vi "RVHR - Coerce Slider.vi"(6 "Local Data in":T1, 7 "UI Refs":T8, 8 "error in (no error)":errorcluster, 11 "New Distance":dbl) -> (0 "error out":errorcluster, 3 "Coerced Distance":dbl, 4 "Local Data out":T1)   [LabVIEW 2024]
uses:
  Controls/RVHR - UI Refs.ctl
  Controls/RVHR - Local Data.ctl
  Controls/Test Cluster.ctl
  Controls/Excluded Information.ctl
  Controls/Language.ctl
  Controls/Device_Type.ctl
  <vilib>/Utility/miscctls.llb/LVRectTypeDef.ctl
  <vilib>/Utility/miscctls.llb/LVBoundsTypeDef.ctl
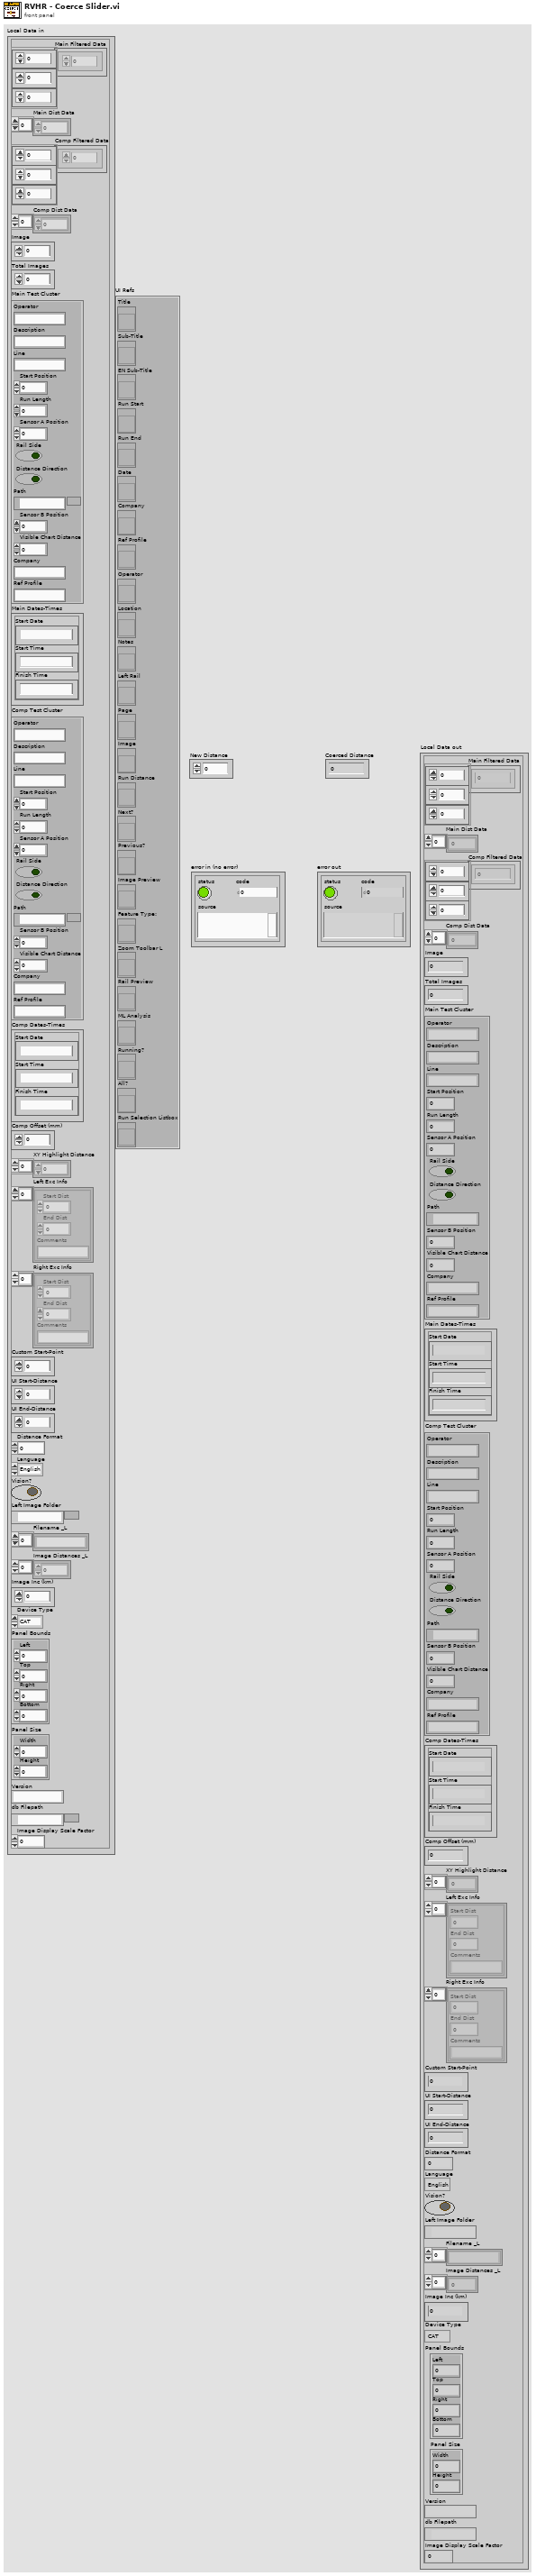
[diagram p1: front panel]
types:
  T1 = typedef "RVHR - Local Data.ctl" = cluster{"Main Filtered Data":dbl[][][], "Main Dist Data":dbl[], "Comp Filtered Data":dbl[][][], "Comp Dist Data":dbl[], "Image":u16, "Total Images":u16, "Main Test Cluster":T2, "Main Dates-Times":cluster{"Start Date":string, "Start Time":string, "Finish Time":string}, "Comp Test Cluster":T2, "Comp Dates-Times":cluster{"Start Date":string, "Start Time":string, "Finish Time":string}, "Comp Offset (mm)":i64, "XY Highlight Distance":dbl[], "Left Exc Info":T3[], "Right Exc Info":T3[], "Custom Start-Point":dbl, "UI Start-Distance":dbl, "UI End-Distance":dbl, "Distance Format":u8, "Language":T4, "Vision?":bool, "Left Image Folder":path, "Filename _L":string[], "Image Distances _L":dbl[], "Image Inc (km)":dbl, "Device Type":T5, "Panel Bounds":T6, "Panel Size":T7, "Version":string, "db Filepath":path, "Image Display Scale Factor":dbl}
  T2 = typedef "Test Cluster.ctl" = cluster{"Operator":string, "Description":string, "Line":string, "Start Position":dbl, "Run Length":dbl, "Sensor A Position":dbl, "Rail Side":bool, "Distance Direction":bool, "Path":path, "Sensor B Position":dbl, "Visible Chart Distance":dbl, "Company":string, "Ref Profile":string}
  T3 = typedef "Excluded Information.ctl" = cluster{"Start Dist":dbl, "End Dist":dbl, "Comments":string}
  T4 = typedef "Language.ctl" = enum16{"English", "Chinese", "German"}
  T5 = typedef "Device_Type.ctl" = enum16{"CAT", "Bi-CAT", "YRCA", "RCA", "RV-HR", "TV-HR"}
  T6 = typedef "LVRectTypeDef.ctl" = cluster{"Left":i16, "Top":i16, "Right":i16, "Bottom":i16}
  T7 = typedef "LVBoundsTypeDef.ctl" = cluster{"Width":u32, "Height":u32}
  T8 = typedef "RVHR - UI Refs.ctl" = cluster{"Title":refnum<vi>, "Sub-Title":refnum<vi>, "EN Sub-Title":refnum<vi>, "Run Start":refnum<vi>, "Run End":refnum<vi>, "Date":refnum<vi>, "Company":refnum<vi>, "Ref Profile":refnum<vi>, "Operator":refnum<vi>, "Location":refnum<vi>, "Notes":refnum<vi>, "Left Rail":refnum<vi>, "Page":refnum<vi>, "Image":refnum<vi>, "Run Distance":refnum<vi>, "Next?":refnum<vi>, "Previous?":refnum<vi>, "Image Preview":refnum<vi>, "Feature Type:":refnum<vi>, "Zoom Toolbar L":refnum<vi>, "Rail Preview":refnum<vi>, "ML Analysis":refnum<vi>, "Running?":refnum<vi>, "All?":refnum<vi>, "Run Selection Listbox":refnum<vi>}
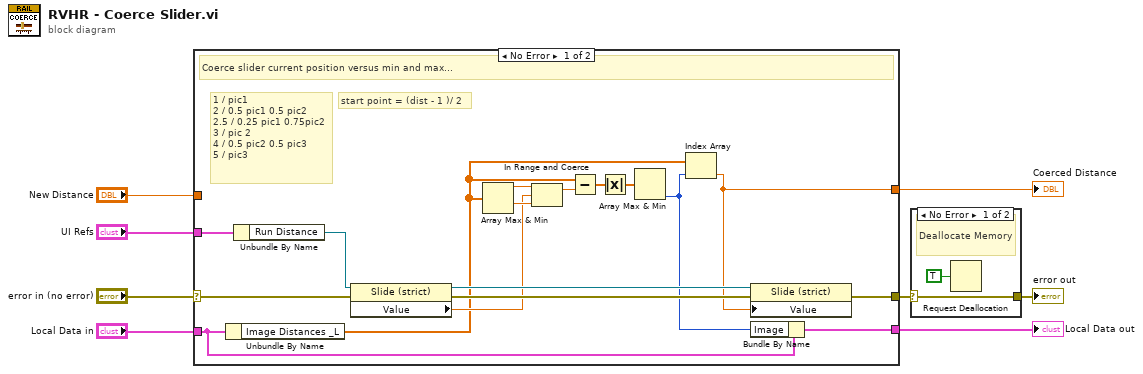
[diagram p0: block diagram]
diagram:
  n1 = case shown="No Error" "error in (no error)" {
    selector: "error in (no error)" -> [w24 w27]
    tunnel: "UI Refs" -> [w25 _]
    tunnel: [w20 w27] -> w3
    tunnel: [w12 _] -> w8
    tunnel: "New Distance" -> [_ _]
    tunnel: "Local Data in" -> [w11 w26]
    tunnel: [w9 w26] -> w1
    frame No Error {
      # "start point = (dist - 1 )/ 2"
      # "1 / pic1\n2 / 0.5 pic1 0.5 pic2\n2.5 / 0.25 pic1 0.75pic2\n3 / pic 2\n4 / 0.5 pic2 0.5 pic3\n5 / pic3"
      # "Coerce slider current position versus min and max..."
      n2 = Unbundle By Name(w11) -> ("Image Distances _L"=w13:dbl[])
      n3 = Unbundle By Name(w25) -> ("Run Distance"=w23:refnum<vi>)
      n4 = property class="Slide (strict)"(reference=w23, error in=w24) -> (reference out=w21:refnum<vi>, error out=w22:errorcluster, "Value"=w17:dbl)
      n5 = Array Max & Min(array=w13) -> (max value=w18:dbl, min value=w19:dbl)  [unwired: 2 out]
      n6 = In Range and Coerce(upper limit=w18, x=w17, lower limit=w19) -> (coerced(x)=w16:dbl)  [unwired: 1 out]
      n7 = Subtract(x=w13, y=w16) -> (x-y=w15:dbl[])
      n8 = Absolute Value(x=w15) -> (abs(x)=w14:dbl[])
      n9 = Array Max & Min(array=w14) -> (min index (indices)=w10:i32)  [unwired: 3 out]
      n10 = Index Array(array=w13, index=w10) -> (element=w12:dbl)
      n11 = property class="Slide (strict)"(reference=w21, error in=w22, "Value"=w12) -> (error out=w20:errorcluster)  [unwired: 1 out]
      n12 = Bundle By Name(cluster=w11, "Image"=w10) -> (w9:T1)
    }
    frame Error {
    }
  }
  "Coerced Distance" <- w8
  "Local Data out" <- w1
  n13 = case shown="No Error" w3 {
    selector: w3 -> [w28 w30]
    tunnel: [w28 w30] -> w2
    frame No Error {
      # "Deallocate Memory"
      n14 = Request Deallocation(TRUE ("flag")) -> ()
    }
    frame Error {
    }
  }
  "error out" <- w2
